vi "Write Strategies.vi"(9 "Strategies.Test":T1, 10 "Strategies.Assert":T2, 11 "Banana in":refnum<class "Banana.lvclass">) -> (3 "Banana out":refnum<class "Banana.lvclass">)   [LabVIEW 2021, in "Bananas.lvlib" / "Banana.lvclass"]
uses:
  Banana.lvclass
  Assertion Strategies -- cluster.ctl
  AssertTrue/AssertTrue.lvclass
  AssertFalse/AssertFalse.lvclass
  Banana.lvclass/Banana.ctl
  Bananas.lvlib
  DefineTest/DefineTest.lvclass
  Test Strategies -- cluster.ctl
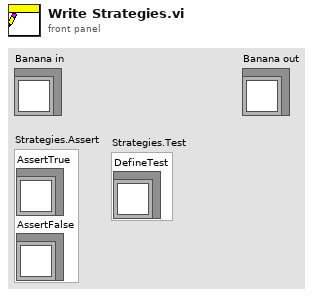
[diagram p1: front panel]
types:
  T1 = typedef "Bananas.lvlib/Test Strategies -- cluster.ctl" = cluster{"DefineTest":refnum<class "DefineTest.lvclass">}
  T2 = typedef "Bananas.lvlib/Assertion Strategies -- cluster.ctl" = cluster{"AssertTrue":refnum<class "AssertTrue.lvclass">, "AssertFalse":refnum<class "AssertFalse.lvclass">}
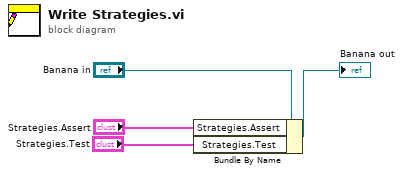
[diagram p0: block diagram]
diagram:
  n1 = Bundle By Name(cluster="Banana in", "Strategies.Assert"="Strategies.Assert", "Strategies.Test"="Strategies.Test") -> (→"Banana out":refnum<class "Banana.lvclass">)
